vi "UnoLoopbackTesterv4.vi"() -> ()   [LabVIEW 2009]
uses:
  <vilib>/Instr/_visa.llb/VISA Configure Serial Port (Instr).vi
panel:
  in  "stop":bool
  in  "System":enum32{"Main", "Serial Terminal"}(tab)=enum."Serial Terminal"
  out "Outgoing Messages":string
  in  "Send":bool
  in  "Input":string
  out "Incoming Messages":string
  in  "VISA resource name":refnum<visa-resource-name>
  in  "baud rate (9600)":u32=9600
  in  "data bits (8)":u16=8 min=5 max=8 step=1
  in  "parity (0:none)":enum16{"None", "Odd", "Even", "Mark", "Space"}(ring)
  in  "stop bits (10: 1 bit)":u16(ring)=10 items=["1.0"=10, "1.5"=15, "2.0"=20]
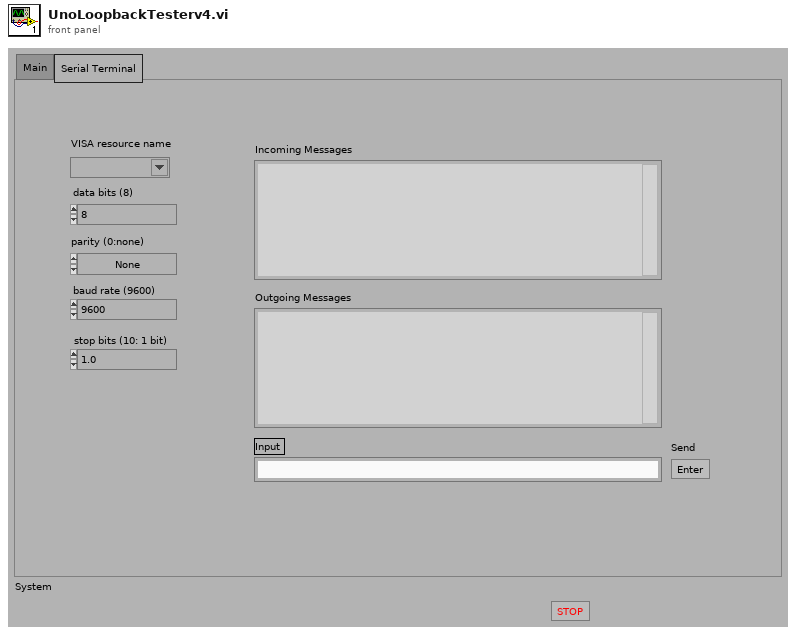
[diagram p1: front panel]
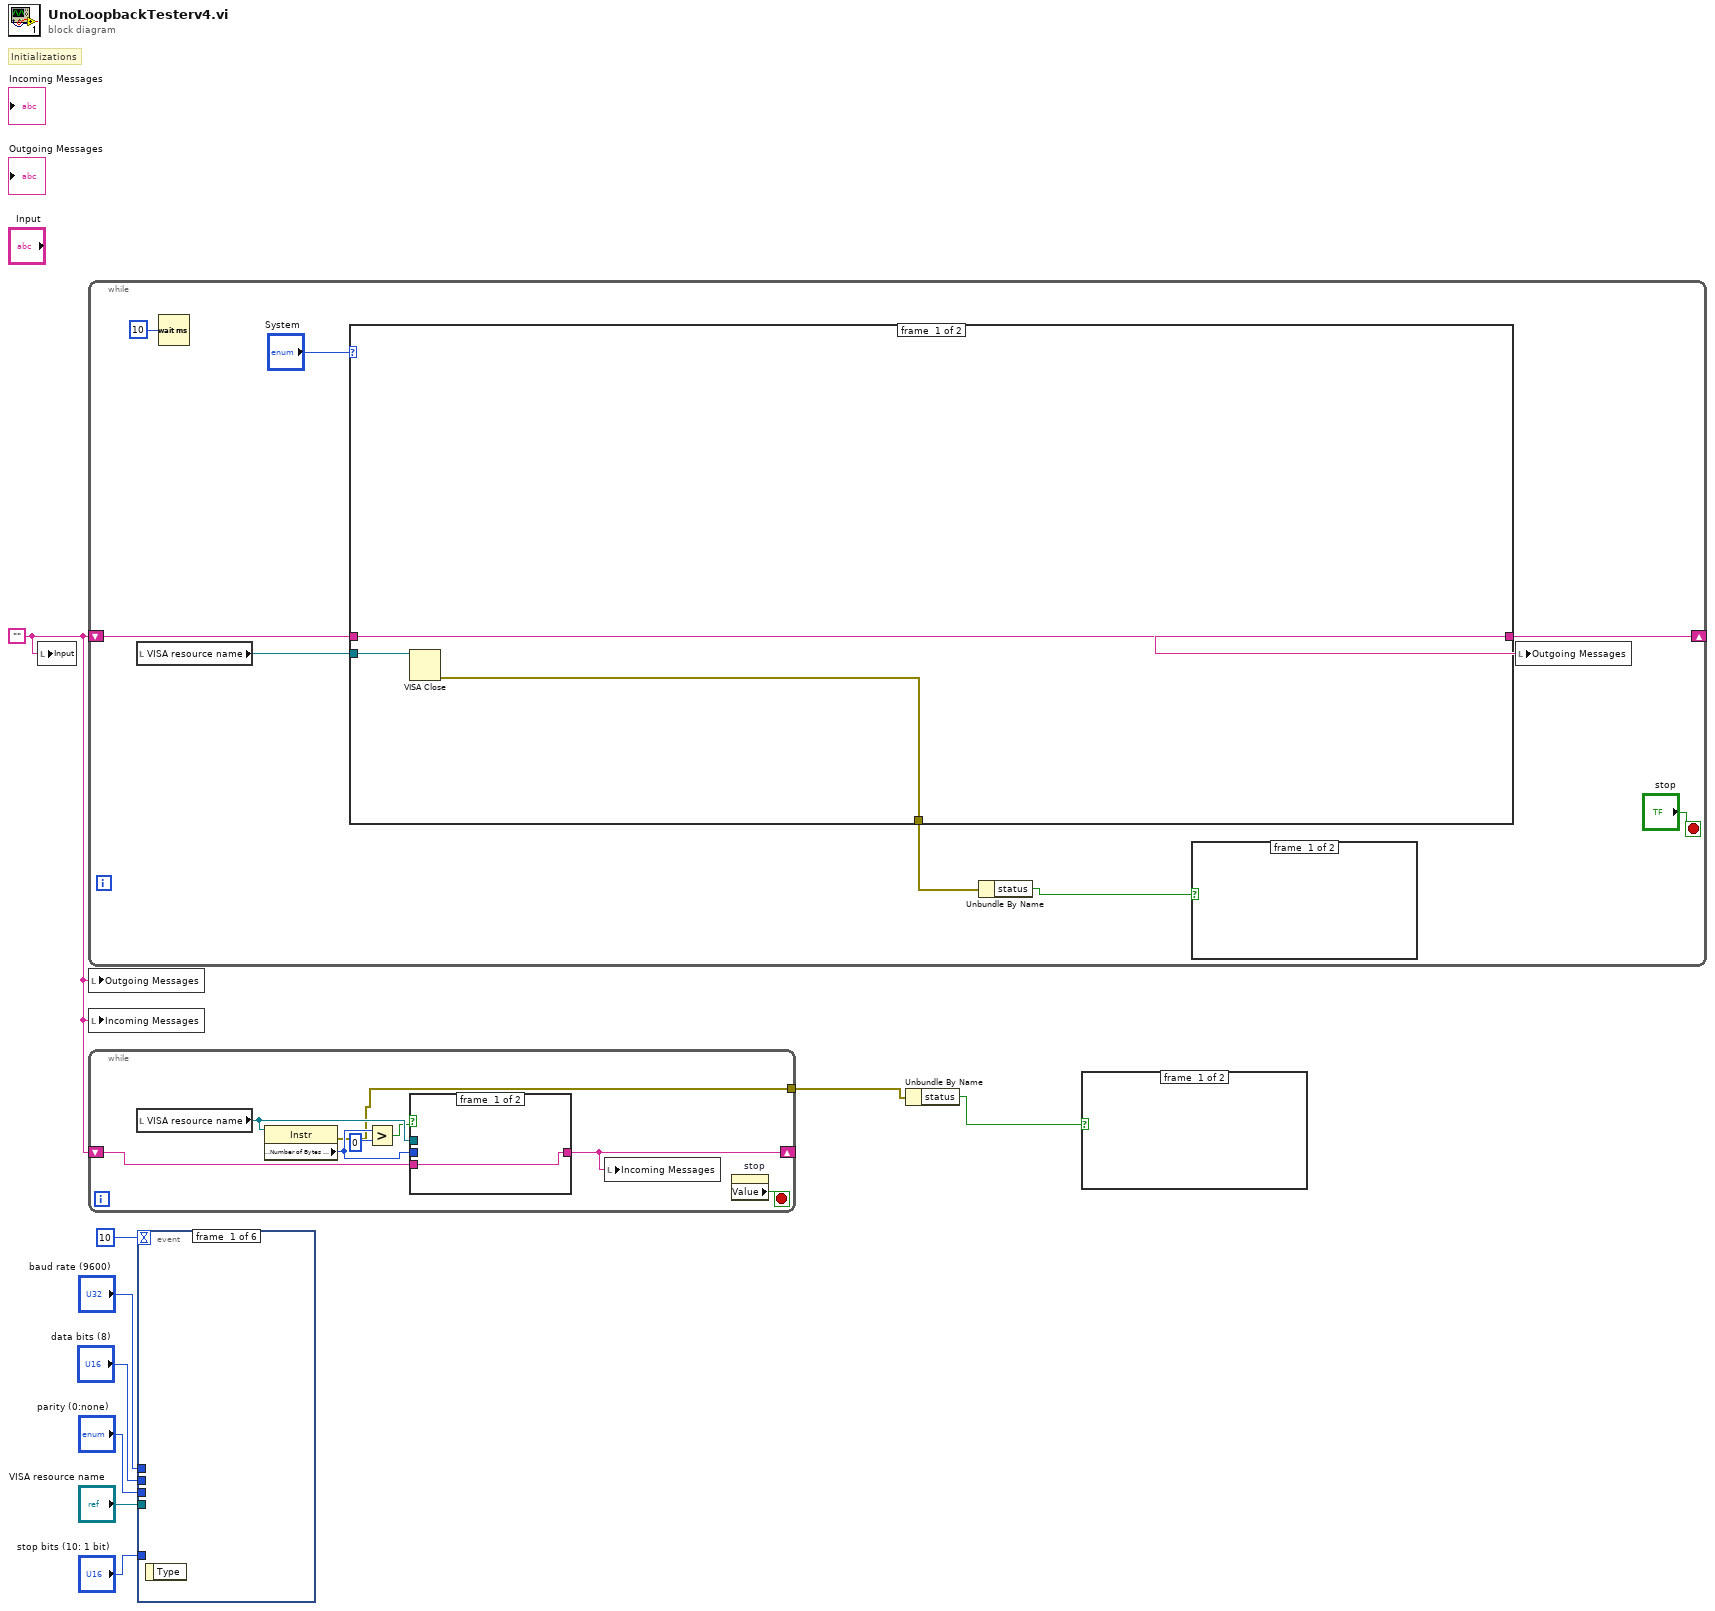
[diagram p0: block diagram]
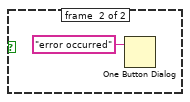
[diagram p2: hidden frame]
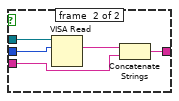
[diagram p3: hidden frame]
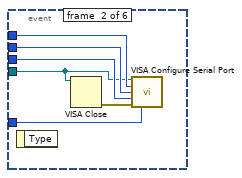
[diagram p4: hidden frame]
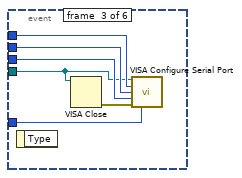
[diagram p5: hidden frame]
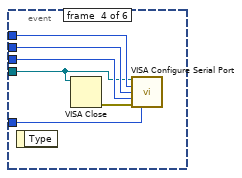
[diagram p6: hidden frame]
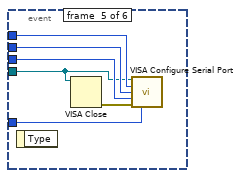
[diagram p7: hidden frame]
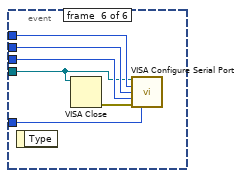
[diagram p8: hidden frame]
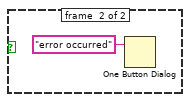
[diagram p9: hidden frame]
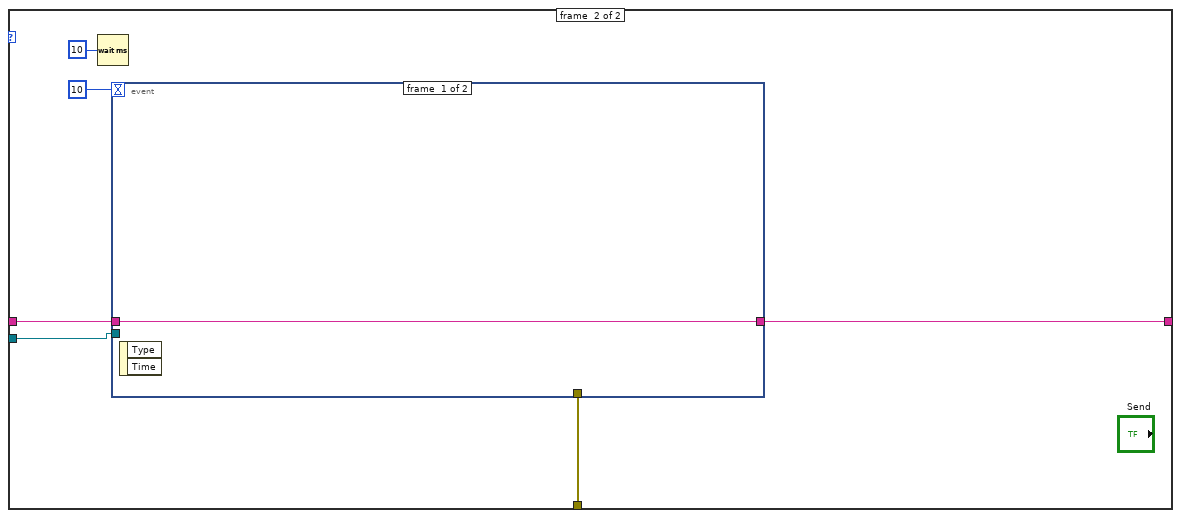
[diagram p10: hidden frame]
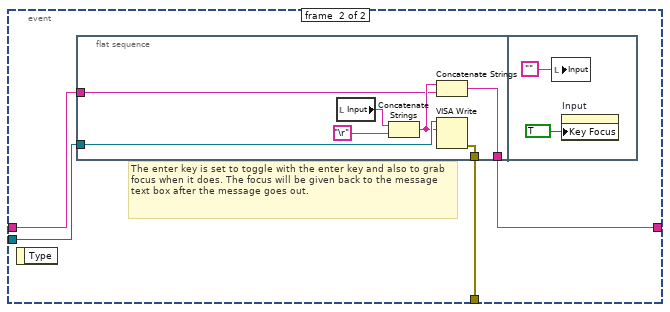
[diagram p11: hidden frame]
diagram:
  w3 = ""
  # "Initializations"
  n1 = local write "Input"(w3) -> ()
  n2 = while {
    shift-right: [w13] -> _
    shift-left: w3 -> [w14]
    stop <- "stop" stop-if-true
    n3 = local read "VISA resource name"() -> (w15:refnum<visa-resource-name>)
    n4 = Wait (ms)(milliseconds to wait=u32 10) -> ()  [unwired: 1 out]
    n5 = case shown="\"Serial Terminal\"" "System" {
      tunnel: w15 -> [w21 w25]
      tunnel: [w20 w24] -> w13
      tunnel: w14 -> [w20 w23]
      tunnel: [w19 w22] -> w11
      frame #0 {
        n6 = VISA Close(VISA resource name=w21) -> (error out=w19:errorcluster)  [unwired: 1 in]
      }
      frame #1 {
        n7 = Wait (ms)(milliseconds to wait=u32 10) -> ()  [unwired: 1 out]
        n8 = event shown="[1] \"Send\": Value Change" {
          selector: _ -> [_ _]
          dyn-events: _ -> [_ _]
          timeout: 10 -> [_ _]
          tunnel: w25 -> [_ w32]
          tunnel: [w28 w30] -> w24
          tunnel: w23 -> [w28 w31]
          tunnel: [_ w29] -> w22
          event #0 {
            n9 = event-data() -> ()  [unwired: 1 in, 2 out]
          }
          event #1 {
            # "The enter key is set to toggle with the enter key and also to grab focus when it does. The focus will be given back to the message text box after the message goes out."
            n10 = event-data() -> ()  [unwired: 1 in, 1 out]
            n11 = flat-sequence {
              tunnel: w32 -> [w37]
              tunnel: w31 -> [w35]
              tunnel: [w34] -> w30
              tunnel: [w33] -> w29
              frame #0 {
                n12 = local read "Input"() -> (w39:string)
                n13 = Concatenate Strings(w39, "\r") -> (w36:string)
                n14 = Concatenate Strings(w36, w35) -> (w34:string)
                n15 = VISA Write(VISA resource name=w37, write buffer=w36) -> (error out=w33:errorcluster)  [unwired: 1 in, 2 out]
              }
              frame #1 {
                n16 = local write "Input"("") -> ()
                n17 = property on="Input" class="Str"("Key Focus"=TRUE) -> ()  [unwired: 2 in, 2 out]
              }
            }
          }
        }
      }
    }
    n18 = Unbundle By Name(w11) -> ("status"=w10:bool)
    n19 = case shown="True" w10 {
      frame #0 {
      }
      frame #1 {
        n20 = One Button Dialog(message="error occurred") -> ()  [unwired: 1 in, 1 out]
      }
    }
    n21 = local write "Outgoing Messages"(w13) -> ()
  }
  n22 = local write "Outgoing Messages"(w3) -> ()
  n23 = local write "Incoming Messages"(w3) -> ()
  n24 = while {
    shift-right: [w43] -> _
    shift-left: w3 -> [w44]
    tunnel: [w42] -> w2
    stop <- w48 stop-if-true
    n25 = local read "VISA resource name"() -> (w49:refnum<visa-resource-name>)
    n26 = property class="Instr"(reference=w49) -> (error out=w42:errorcluster, "Serial Settings:Number of Bytes at Serial Port"=w45:u32)  [unwired: 1 in, 1 out]
    n27 = Greater?(x=w45, y=u32 0) -> (0:w46:bool)
    n28 = case shown="False" w46 {
      tunnel: w49 -> [_ w55]
      tunnel: w45 -> [_ w54]
      tunnel: w44 -> [w50 w51]
      tunnel: [w50 w52] -> w43
      frame #0 {
      }
      frame #1 {
        n29 = VISA Read(VISA resource name=w55, byte count=w54) -> (read buffer=w53:string)  [unwired: 1 in, 3 out]
        n30 = Concatenate Strings(w53, w51) -> (w52:string)
      }
    }
    n31 = local write "Incoming Messages"(w43) -> ()
    n32 = property on="stop" class="Bool (strict)"() -> ("Value"=w48:bool)  [unwired: 2 in, 2 out]
  }
  n33 = event shown="[5] \"stop bits (10: 1 bit)\": Value Change" {
    selector: _ -> [_ _ _ _ _ _]
    dyn-events: _ -> [_ _ _ _ _ _]
    timeout: 10 -> [_ _ _ _ _ _]
    tunnel: "VISA resource name" -> [_ w56 w62 w68 w74 w80]
    tunnel: "baud rate (9600)" -> [_ w61 w67 w73 w79 w85]
    tunnel: "data bits (8)" -> [_ w60 w66 w72 w78 w84]
    tunnel: "parity (0:none)" -> [_ w59 w65 w71 w77 w83]
    tunnel: "stop bits (10: 1 bit)" -> [_ w58 w64 w70 w76 w82]
    event #0 {
      n34 = event-data() -> ()  [unwired: 1 in, 1 out]
    }
    event #1 {
      n35 = event-data() -> ()  [unwired: 1 in, 1 out]
      n36 = VISA Close(VISA resource name=w56) -> (error out=w57:errorcluster)  [unwired: 1 in]
      n37 = call-poly "VISA Configure Serial Port"("VISA resource name"=w56, "baud rate (9600)"=w61, "data bits (8)"=w60, "parity (0:none)"=w59, "error in (no error)"=w57, "stop bits (10: 1 bit)"=w58) -> ()  [unwired: 8 in, 2 out]
    }
    event #2 {
      n38 = event-data() -> ()  [unwired: 1 in, 1 out]
      n39 = VISA Close(VISA resource name=w62) -> (error out=w63:errorcluster)  [unwired: 1 in]
      n40 = call-poly "VISA Configure Serial Port"("VISA resource name"=w62, "baud rate (9600)"=w67, "data bits (8)"=w66, "parity (0:none)"=w65, "error in (no error)"=w63, "stop bits (10: 1 bit)"=w64) -> ()  [unwired: 8 in, 2 out]
    }
    event #3 {
      n41 = event-data() -> ()  [unwired: 1 in, 1 out]
      n42 = VISA Close(VISA resource name=w68) -> (error out=w69:errorcluster)  [unwired: 1 in]
      n43 = call-poly "VISA Configure Serial Port"("VISA resource name"=w68, "baud rate (9600)"=w73, "data bits (8)"=w72, "parity (0:none)"=w71, "error in (no error)"=w69, "stop bits (10: 1 bit)"=w70) -> ()  [unwired: 8 in, 2 out]
    }
    event #4 {
      n44 = event-data() -> ()  [unwired: 1 in, 1 out]
      n45 = VISA Close(VISA resource name=w74) -> (error out=w75:errorcluster)  [unwired: 1 in]
      n46 = call-poly "VISA Configure Serial Port"("VISA resource name"=w74, "baud rate (9600)"=w79, "data bits (8)"=w78, "parity (0:none)"=w77, "error in (no error)"=w75, "stop bits (10: 1 bit)"=w76) -> ()  [unwired: 8 in, 2 out]
    }
    event #5 {
      n47 = event-data() -> ()  [unwired: 1 in, 1 out]
      n48 = VISA Close(VISA resource name=w80) -> (error out=w81:errorcluster)  [unwired: 1 in]
      n49 = call-poly "VISA Configure Serial Port"("VISA resource name"=w80, "baud rate (9600)"=w85, "data bits (8)"=w84, "parity (0:none)"=w83, "error in (no error)"=w81, "stop bits (10: 1 bit)"=w82) -> ()  [unwired: 8 in, 2 out]
    }
  }
  n50 = Unbundle By Name(w2) -> ("status"=w1:bool)
  n51 = case shown="True" w1 {
    frame #0 {
    }
    frame #1 {
      n52 = One Button Dialog(message="error occurred") -> ()  [unwired: 1 in, 1 out]
    }
  }
